vi "read_txt.vi"(10 "file_path":path, 11 "IntensityGraph in":refnum<vi>) -> (1 "image_info":T1, 2 "step_size_V":dbl, 3 "image":dbl[][](array[numeric]))   [LabVIEW 2014]
uses:
  <vilib>/Utility/file.llb/Read From Spreadsheet File (string).vi
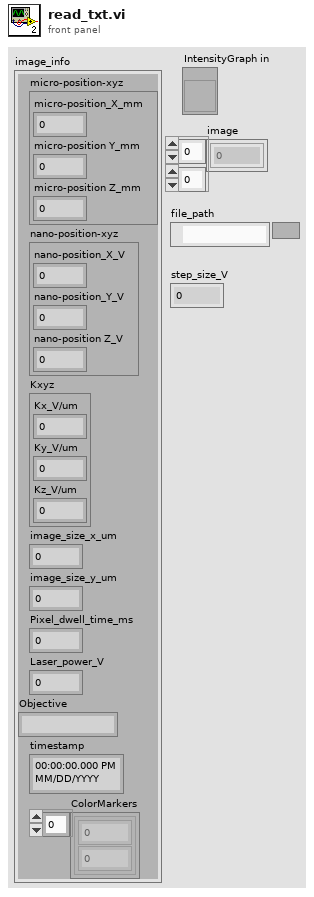
[diagram p1: front panel]
types:
  T1 = cluster{"micro-position-xyz":cluster{"micro-position_X_mm":sgl, "micro-position Y_mm":sgl, "micro-position Z_mm":sgl}, "nano-position-xyz":cluster{"nano-position_X_V":sgl, "nano-position_Y_V":sgl, "nano-position Z_V":sgl}, "Kxyz":cluster{"Kx_V/um":sgl, "Ky_V/um":sgl, "Kz_V/um":sgl}, "image_size_x_um":sgl, "image_size_y_um":sgl, "Pixel_dwell_time_ms":sgl, "Laser_power_V":sgl, "Objective":string, "timestamp":timestamp, "ColorMarkers":cluster{dbl, u32}[]}
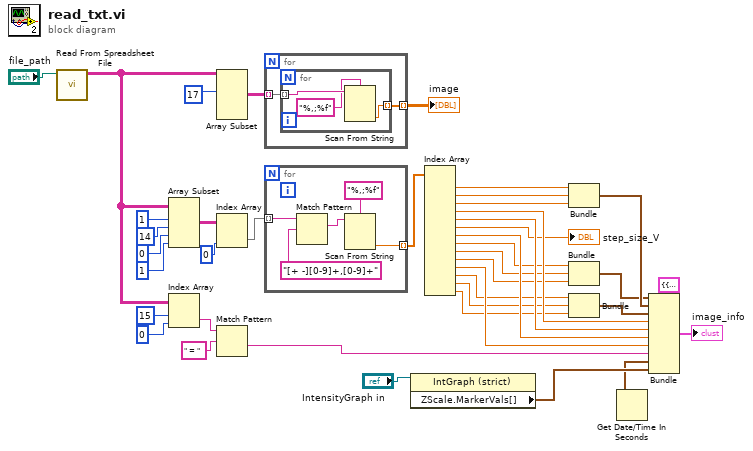
[diagram p0: block diagram]
diagram:
  n1 = call-poly <vilib>:"Read From Spreadsheet File.vi"("file path (dialog if empty)"="file_path") -> ("all rows"=w15:string[][])  [unwired: 6 in, 4 out]
  n2 = Array Subset(array=w15, index (row)=1 ("index"), length (row)=14 ("length"), index (col)=0 ("index"), length (col)=1 ("length")) -> (w9:string[][])
  n3 = Index Array(array=w15, index (row)=15, index (col)=0 ("disabled index (col)")) -> (element=w18:string)
  n4 = Array Subset(array=w15, index (row)=17 ("index")) -> (w4:string[][])  [unwired: 3 in]
  n5 = Index Array(array=w9, index (col)=0 ("disabled index (col)")) -> (element=w10:string[])  [unwired: 1 in]
  n6 = Match Pattern(string=w18, regular expression=" = ") -> (after substring=w33:string)  [unwired: 1 in, 3 out]
  n7 = for {
    tunnel: w4 -> [w42] mode=indexing
    tunnel: [w41] -> w5 mode=indexing
    n8 = for {
      tunnel: w42 -> [w45] mode=indexing
      tunnel: [w44] -> w41 mode=indexing
      n9 = Scan From String(format string="%,;%f", input string=w45) -> (output 1=w44:dbl)  [unwired: 3 in, 3 out]
    }
  }
  "image" <- w5
  n10 = for {
    tunnel: w10 -> [w50] mode=indexing
    tunnel: [w46] -> w13 mode=indexing
    n11 = Match Pattern(string=w50, regular expression="[+ -][0-9]+,[0-9]+") -> (match substring=w48:string)  [unwired: 1 in, 3 out]
    n12 = Scan From String(format string="%,;%f", input string=w48) -> (output 1=w46:dbl)  [unwired: 3 in, 3 out]
  }
  n13 = property on="Property Node" class="IntGraph (strict)"(reference="IntensityGraph in") -> ("ZScale.MarkerVals[]"=w35:cluster{dbl, u32}[])  [unwired: 1 in, 2 out]
  n14 = Index Array(array=w13) -> (element #1=w28:dbl, element #2=w29:dbl, element #3=w30:dbl, element #4=w39:dbl, element #5=w38:dbl, element #6=→"step_size_V":dbl, element #7=w37:dbl, element #8=w23:dbl, element #9=w24:dbl, element #10=w25:dbl, element #11=w36:dbl, element #12=w22:dbl, element #13=w21:dbl, element #14=w20:dbl)  [unwired: 14 in]
  n15 = Bundle(w28, w29, w30) -> (w31:cluster{dbl, dbl, dbl})  [unwired: 1 in]
  n16 = Bundle(w23, w24, w25) -> (w27:cluster{dbl, dbl, dbl})  [unwired: 1 in]
  n17 = Bundle(w22, w21, w20) -> (w32:cluster{dbl, dbl, dbl})  [unwired: 1 in]
  n18 = Get Date/Time In Seconds() -> (seconds since 1Jan1904=w34:timestamp)
  n19 = Bundle(cluster=T1 {"micro-position-xyz"={"micro-position_X_mm"=1.0, "micro-position Y_mm"=1.0, "micro-position Z_mm"=1.0}, "nano-position-xyz"={"nano-position_X_V"=1.0, "nano-position_Y_V"=1.0, "nano-position Z_V"=1.0}, "Kxyz"={"Kx_V/um"=1.0, "Ky_V/um"=1.0, "Kz_V/um"=1.0}, "image_size_x_um"=1.0, "image_size_y_um"=1.0, "Pixel_dwell_time_ms"=1.0, "Laser_power_V"=1.0, "Objective"="", "timestamp"=timestamp(0 s since 1904-01-01), "ColorMarkers"=[]} ("Image_info"), "micro-position-xyz"=w27, "nano-position-xyz"=w31, "Kxyz"=w32, "image_size_x_um"=w39, "image_size_y_um"=w38, "Pixel_dwell_time_ms"=w37, "Laser_power_V"=w36, "Objective"=w33, "timestamp"=w34, "ColorMarkers"=w35) -> (→"image_info":T1)
